vi "Write Channel List.vi"(8 "error in (no error)":errorcluster, 10 "Channel List":refnum<class "HK Item.lvclass">[](array[class]), 11 "Temp Control in":refnum<class "Temp Control.lvclass">) -> (0 "error out":errorcluster, 3 "Temp Control out":refnum<class "Temp Control.lvclass">)   [LabVIEW 2022 SP3, in "Temp Control.lvclass"]
uses:
  Temp Control.lvclass
  Temp Control.lvclass/Temp Control.ctl
  hk-channel-class/hk-channel-class/HK Item/HK Item.lvclass
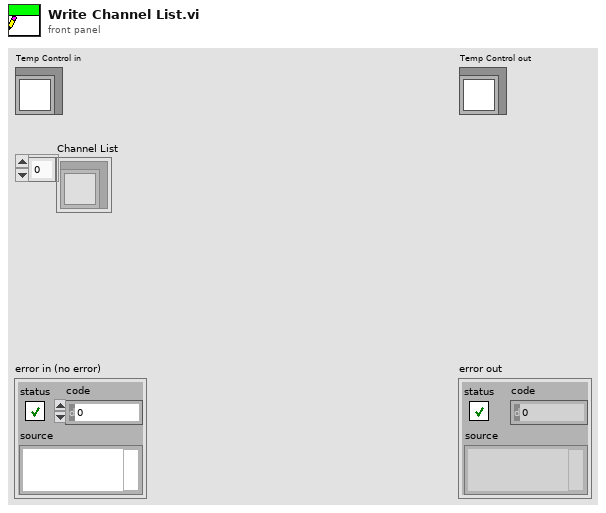
[diagram p1: front panel]
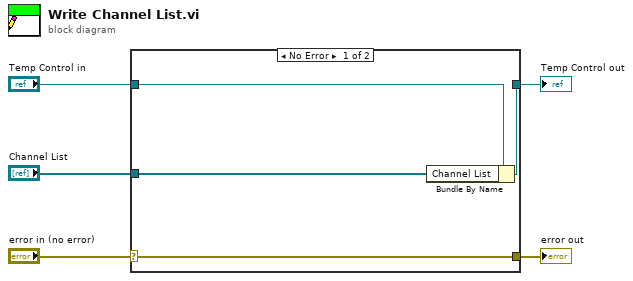
[diagram p0: block diagram]
diagram:
  n1 = case shown="No Error" "error in (no error)" {
    selector: "error in (no error)" -> [w9 w10]
    tunnel: [w9 w10] -> w4
    tunnel: [w7 w11] -> w2
    tunnel: "Temp Control in" -> [w8 w11]
    tunnel: "Channel List" -> [w6 _]
    frame No Error {
      n2 = Bundle By Name(cluster=w8, "Channel List"=w6) -> (w7:refnum<class "Temp Control.lvclass">)
    }
    frame Error {
    }
  }
  "error out" <- w4
  "Temp Control out" <- w2
